vi "Calib_Ref_info.vi"(5 "Input string":string, 6 "Reference Name":string="Instrument to calibrate") -> (0 "Device":string, 1 "Ref Instrument type":T1=enum."Generic Polynomial", 2 "Calib filename":path, 3 "Ch No":i16, 4 "Port":string)   [LabVIEW 2021]
uses:
  Controls/Ref_Inst_type.ctl
panel:
  in  "Ref Instrument type example":T1=enum."Generic Linear"
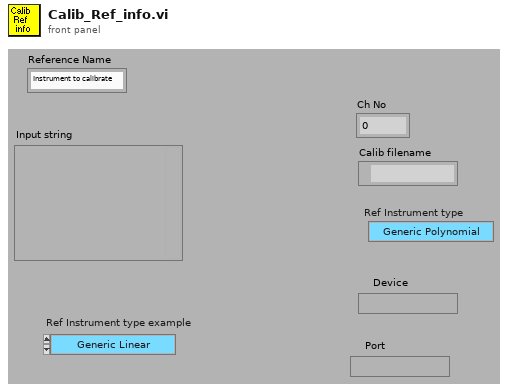
[diagram p1: front panel]
types:
  T1 = typedef "Ref_Inst_type.ctl" = enum16{"Propellor anemometer", "Pressure Transducer", "Raw voltage", "Pitot-static tube", "Generic Linear", "Generic Polynomial", "Thermocouple", "LDA", "Enter Value", "ADAM Channel"}
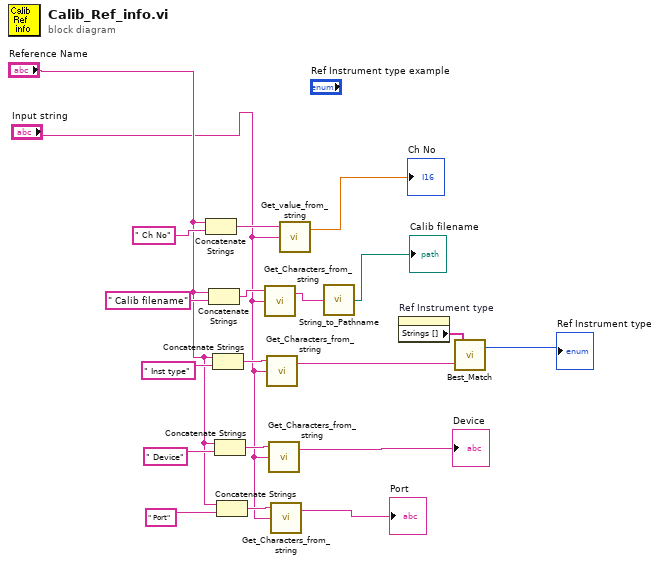
[diagram p0: block diagram]
diagram:
  n1 = Concatenate Strings("Reference Name", " Ch No") -> (w17:string)
  n2 = Concatenate Strings("Reference Name", " Calib filename") -> (w14:string)
  n3 = Concatenate Strings("Reference Name", " Inst type") -> (w12:string)
  n4 = Concatenate Strings("Reference Name", " Device") -> (w11:string)
  n5 = Concatenate Strings("Reference Name", " Port") -> (w4:string)
  n6 = call "Get_Characters_from_string.vi"("Input string"="Input string", "Variable name"=w14) -> ("Value"=w13:string)  [unwired: 1 in, 1 out]
  n7 = call "Get_Characters_from_string.vi"("Input string"="Input string", "Variable name"=w12) -> ("Value"=w19:string)  [unwired: 1 in, 1 out]
  n8 = call "Get_Characters_from_string.vi"("Input string"="Input string", "Variable name"=w11) -> ("Value"=→"Device":string)  [unwired: 1 in, 1 out]
  n9 = call "Get_Characters_from_string.vi"("Input string"="Input string", "Variable name"=w4) -> ("Value"=→"Port":string)  [unwired: 1 in, 1 out]
  n10 = call "Get_value_from_string.vi"("Input string"="Input string", "Variable name"=w17) -> ("Value"=→"Ch No":dbl)  [unwired: 1 in, 1 out]
  n11 = call "String_to_Pathname.vi"("Input String"=w13) -> ("path"=→"Calib filename":path)
  n12 = property on="Ref Instrument type" class="Enum (strict)"() -> ("Strings []"=w20:string[])  [unwired: 2 in, 2 out]
  n13 = call "Best_Match.vi"("Input String"=w19, "String Options"=w20) -> ("index of element"=→"Ref Instrument type":i32)  [unwired: 1 out]
